vi "Eat.vi"(8 "error in (no error)":errorcluster caption="错误输入（无错误）", 10 "字符串":string, 11 "Eat 输入":refnum<class "Eat.lvclass">) -> (0 "error out":errorcluster caption="错误输出", 2 "字符串 2":string, 3 "Eat 输出":refnum<class "Eat.lvclass">)   [LabVIEW 2020, in "Eat.lvclass"]
uses:
  Eat.lvclass
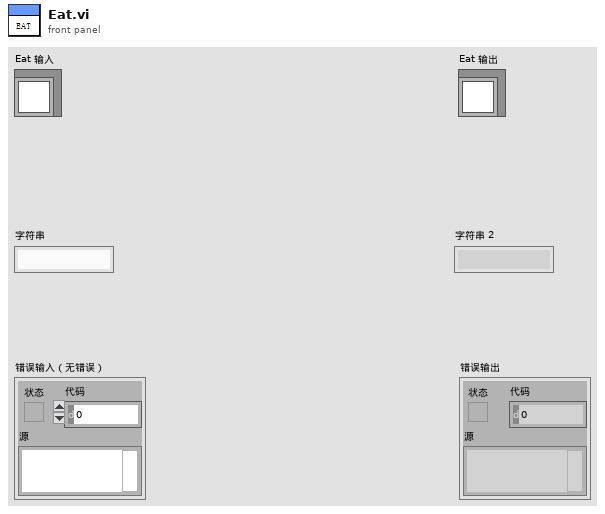
[diagram p1: front panel]
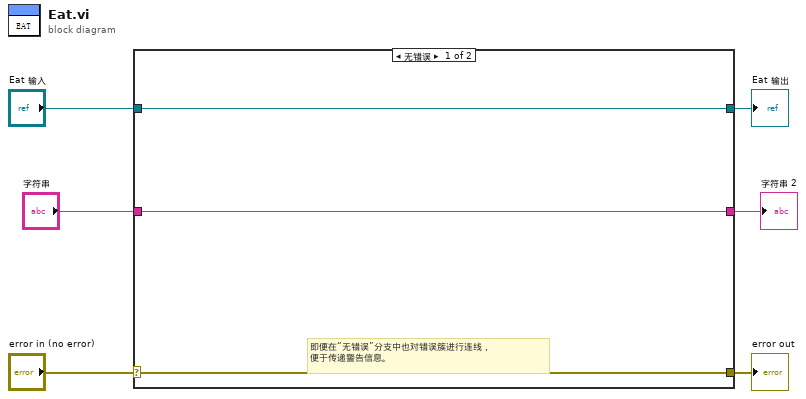
[diagram p0: block diagram]
diagram:
  n1 = case shown="无错误" "error in (no error)" {
    selector: "error in (no error)" -> [w8 w11]
    tunnel: [w8 w11] -> w5
    tunnel: [w9 w10] -> w3
    tunnel: "Eat 输入" -> [w9 w10]
    tunnel: [w7 _] -> w2
    tunnel: "字符串" -> [w7 _]
    frame No Error {
      # "即便在“无错误”分支中也对错误簇进行连线，\n便于传递警告信息。"
    }
    frame Error {
    }
  }
  "error out" <- w5
  "Eat 输出" <- w3
  "字符串 2" <- w2
